vi "front_panel.vi"() -> ()   [LabVIEW 2020]
uses:
  State control.ctl
panel:
  out "Name 2":string
  out "Comments":string
  out "Process":T1
  in  "Status":T2 {"Status - camera" scale=0.0..10.0; "Status - computer" scale=0.0..10.0; "Status - TV" scale=0.0..10.0; "Status - kettle" scale=0.0..10.0; "Status -  microwave" scale=0.0..10.0; "Status - vacuum cleaner" scale=0.0..10.0; "Status - Fridge" scale=0.0..10.0; "Status - washing machine" scale=0.0..10.0}
  in  "Order":T3
  in  "stop":bool
  in  "Adress":string
  in  "Name":string
  in  "OK Button":bool
  # "ORDER"
  # "Warehouse"
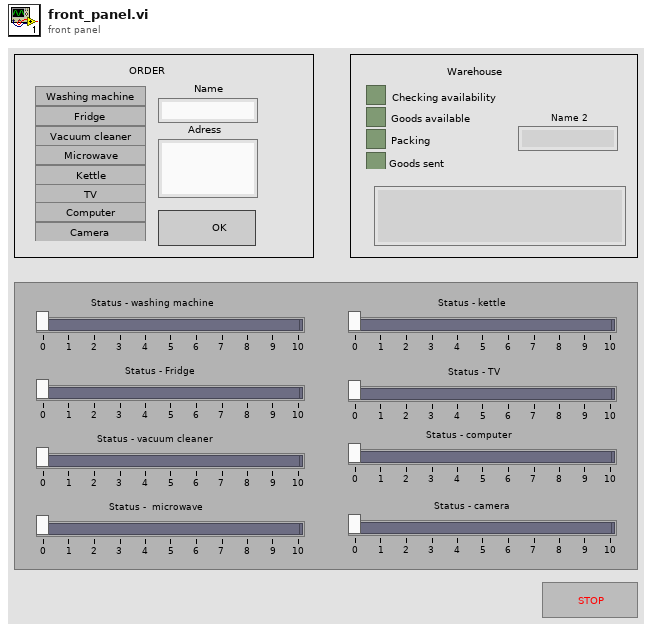
[diagram p1: front panel]
types:
  T1 = cluster{"Checking availability":bool, "Goods available":bool, "Packing":bool, "Goods sent":bool}
  T2 = cluster{"Status - washing machine":u32, "Status - Fridge":u32, "Status - vacuum cleaner":u32, "Status -  microwave":u32, "Status - kettle":u32, "Status - TV":u32, "Status - computer":u32, "Status - camera":u32}
  T3 = cluster{"Washing machine":bool, "Fridge":bool, "Vacuum cleaner":bool, "Microwave":bool, "Kettle":bool, "TV":bool, "Computer":bool, "Camera":bool}
  T4 = typedef "State control.ctl" = enum16{"Init", "avaliability", "goods avaliable", "packing", "sent", "end"}
  T5 = cluster{"Order":cluster{"Washing machine":bool, "Fridge":bool, "Vacuum cleaner":bool, "Microwave":bool, "Kettle":bool, "TV":bool, "Computer":bool, "Camera":bool}, "Adress":string, "Name":string, T4}
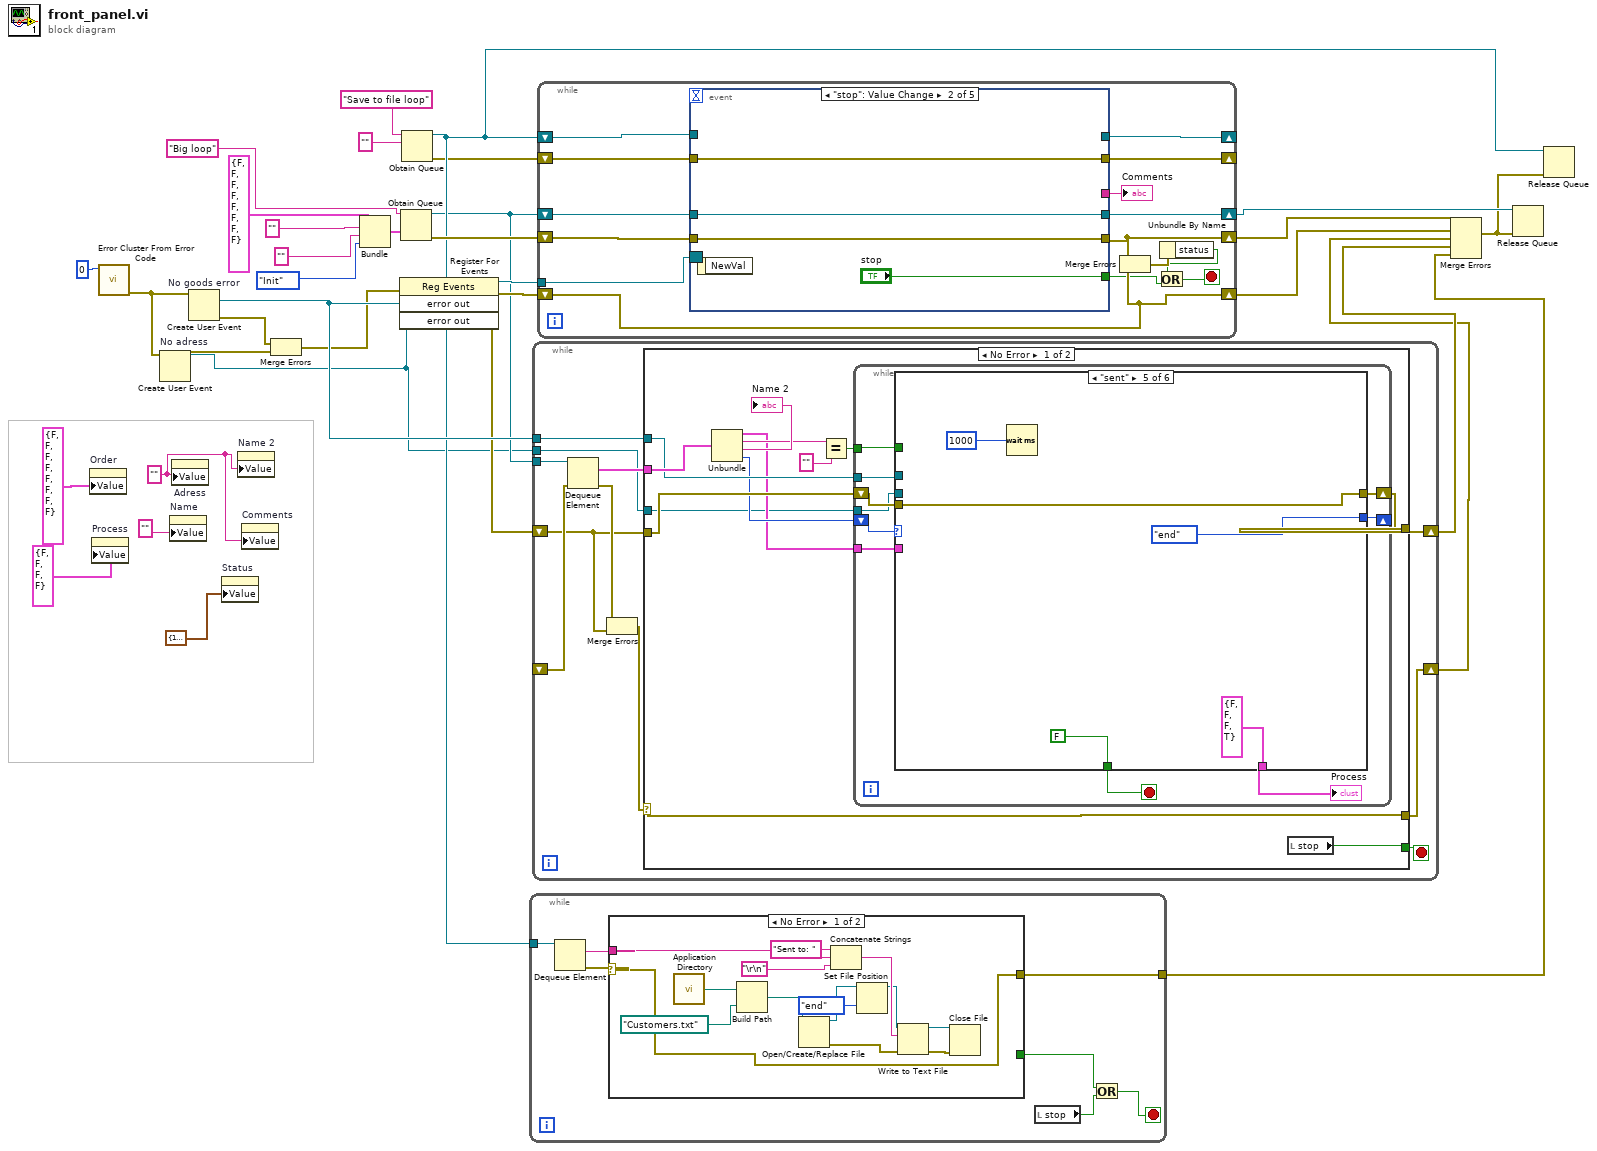
[diagram p0: block diagram]
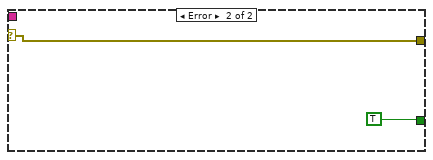
[diagram p2: hidden frame]
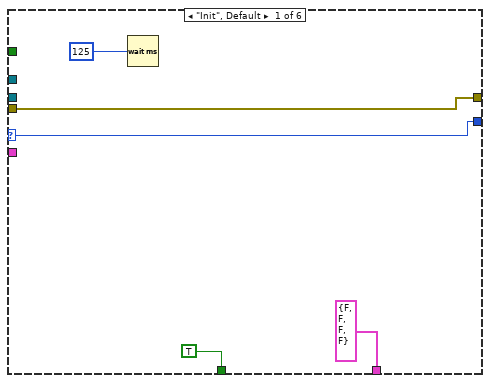
[diagram p3: hidden frame]
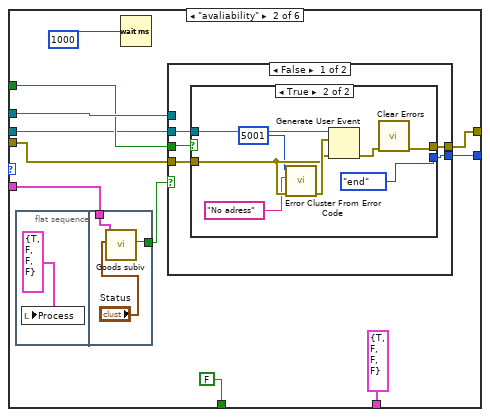
[diagram p4: hidden frame]
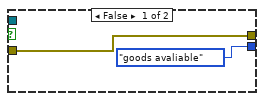
[diagram p5: hidden frame]
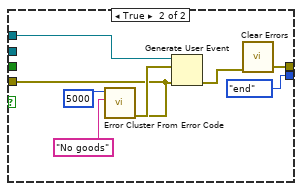
[diagram p6: hidden frame]
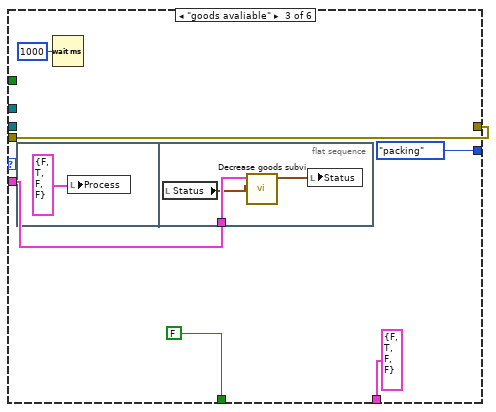
[diagram p7: hidden frame]
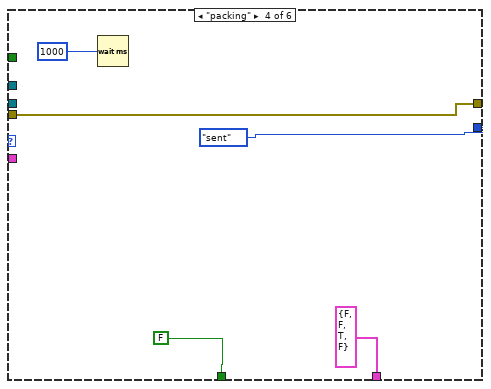
[diagram p8: hidden frame]
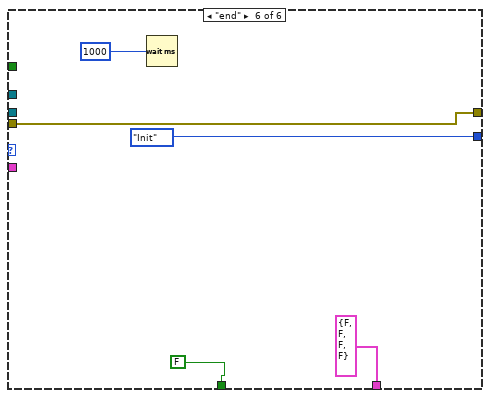
[diagram p9: hidden frame]
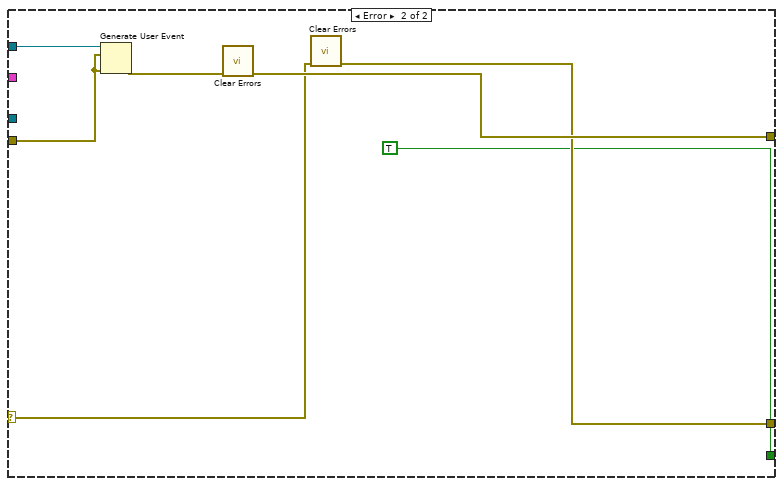
[diagram p10: hidden frame]
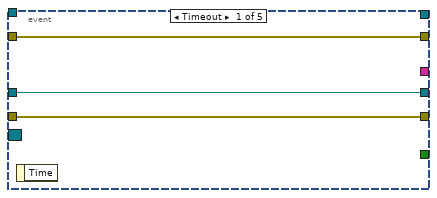
[diagram p11: hidden frame]
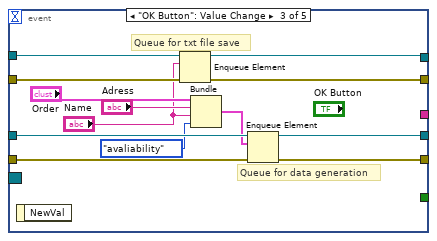
[diagram p12: hidden frame]
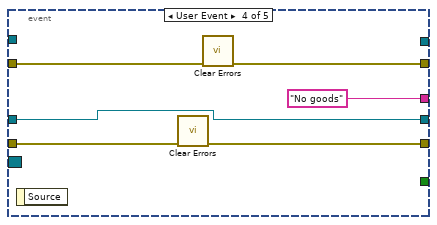
[diagram p13: hidden frame]
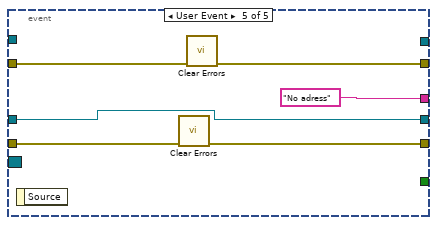
[diagram p14: hidden frame]
diagram:
  w19 = "" ("Adress")
  n1 = property on="Order" class="Clust (strict)"("Value"=T3 {"Washing machine"=FALSE, "Fridge"=FALSE, "Vacuum cleaner"=FALSE, "Microwave"=FALSE, "Kettle"=FALSE, "TV"=FALSE, "Computer"=FALSE, "Camera"=FALSE} ("Order")) -> ()  [unwired: 2 in, 2 out]
  n2 = property on="Process" class="Clust (strict)"("Value"=T1 {"Checking availability"=FALSE, "Goods available"=FALSE, "Packing"=FALSE, "Goods sent"=FALSE} ("Process")) -> ()  [unwired: 2 in, 2 out]
  n3 = call <vilib>:"Error Cluster From Error Code.vi"("error code (0)"=0) -> ("error out"=w9:errorcluster)  [unwired: 8 in]
  n4 = Create User Event "No adress"(user event datatype=w9) -> (user event=w5:refnum<user-event>, error out=w8:errorcluster)  [unwired: 1 in]
  n5 = property on="Name" class="Str"("Value"="" ("Name")) -> ()  [unwired: 2 in, 2 out]
  n6 = property on="Adress" class="Str"("Value"=w19) -> ()  [unwired: 2 in, 2 out]
  n7 = Create User Event "No goods error"(user event datatype=w9) -> (user event=w31:refnum<user-event>, error out=w7:errorcluster)  [unwired: 1 in]
  n8 = property on="Status" class="Clust (strict)"("Value"=T2 {"Status - washing machine"=10, "Status - Fridge"=10, "Status - vacuum cleaner"=10, "Status -  microwave"=10, "Status - kettle"=10, "Status - TV"=10, "Status - computer"=10, "Status - camera"=10} ("Status")) -> ()  [unwired: 2 in, 2 out]
  n9 = property on="Name 2" class="Str"("Value"=w19) -> ()  [unwired: 2 in, 2 out]
  n10 = property on="Comments" class="Str"("Value"=w19) -> ()  [unwired: 2 in, 2 out]
  n11 = Merge Errors(w7, w8) -> (w6:errorcluster)
  n12 = Bundle("Order"=T3 {"Washing machine"=FALSE, "Fridge"=FALSE, "Vacuum cleaner"=FALSE, "Microwave"=FALSE, "Kettle"=FALSE, "TV"=FALSE, "Computer"=FALSE, "Camera"=FALSE}, "Adress"="", "Name"="", State_control."Init") -> (w26:T5)  [unwired: 1 in]
  n13 = register-events(error in=w6, w31, w5) -> (reference out=w32:refnum<event-registration>, error out=w29:errorcluster)  [unwired: 1 in]
  n14 = Obtain Queue(name (unnamed)="Big loop", element data type=w26) -> (queue out=w11:refnum<queue>, error out=w33:errorcluster)  [unwired: 3 in, 1 out]
  n15 = Obtain Queue(name (unnamed)="Save to file loop", element data type="") -> (queue out=w14:refnum<queue>, error out=w13:errorcluster)  [unwired: 3 in, 1 out]
  n16 = while {
    tunnel: w14 -> [w40]
    tunnel: [w34] -> w12
    stop <- w35 stop-if-true
    n17 = Dequeue Element(queue=w40) -> (element=w38:string, error out=w39:errorcluster)  [unwired: 2 in, 2 out]
    n18 = case shown="No Error" w39 {
      selector: w39 -> [w50 w55]
      tunnel: w38 -> [w52 _]
      tunnel: [_ TRUE ("stop")] -> w37
      tunnel: [w50 w55] -> w34
      frame No Error {
        n19 = call <vilib>:"Application Directory.vi"() -> ("Application Directory"=w54:path)
        n20 = Build Path(base path=w54, name or relative path=path "Customers.txt") -> (appended path=w46:path)
        n21 = Open/Create/Replace File(file path (use dialog)=w46) -> (refnum out=w44:refnum<file>, error out=w48:errorcluster)  [unwired: 5 in, 1 out]
        n22 = Concatenate Strings("Sent to: " ("string"), w52, "\r\n") -> (w51:string)
        n23 = Set File Position(refnum=w44, from (0:start)=enum16{"start", "end", "current"}."end") -> (refnum out=w43:refnum<file>)  [unwired: 2 in, 1 out]
        n24 = Write to Text File(file (use dialog)=w43, text=w51, error in=w48) -> (refnum out=w53:refnum<file>, error out=w47:errorcluster)  [unwired: 1 in, 1 out]
        n25 = Close File(refnum=w53, error in=w47) -> ()  [unwired: 2 out]
      }
      frame Error {
      }
    }
    n26 = local read "stop"() -> (w36:bool)
    n27 = Or(x=w37, y=w36) -> (x .or. y?=w35:bool)
  }
  n28 = while {
    tunnel: w11 -> [w67]
    tunnel: w31 -> [w65]
    shift-right: [w59] -> w21
    shift-left: _ -> [w63]
    shift-right: [w62] -> w30
    shift-left: w29 -> [w61]
    tunnel: w5 -> [w57]
    stop <- w58 stop-if-true
    n29 = Dequeue Element(queue=w67, error in (no error)=w63) -> (element=w66:T5, error out=w64:errorcluster)  [unwired: 1 in, 2 out]
    n30 = Merge Errors(w64, w61) -> (w60:errorcluster)
    n31 = case shown="No Error" w60 {
      selector: w60 -> [w80 w161]
      tunnel: w66 -> [w79 _]
      tunnel: w65 -> [w72 w165]
      tunnel: [w73 w162] -> w62
      tunnel: w61 -> [w71 w164]
      tunnel: [w80 w160] -> w59
      tunnel: [w77 TRUE] -> w58
      tunnel: w57 -> [w68 _]
      frame No Error {
        n32 = Unbundle(w79) -> ("Order"=w69:T3, "Adress"=w76:string, "Name"=→"Name 2":string, w70:T4)
        n33 = Equal?(x=w76, y="") -> (x = y?=w74:bool)
        n34 = while {
          tunnel: w74 -> [w89]
          tunnel: w72 -> [w87]
          tunnel: w69 -> [w84]
          shift-right: [w88] -> w73
          shift-left: w71 -> [w86]
          shift-right: [w90] -> _
          shift-left: w70 -> [w85]
          tunnel: w68 -> [w81]
          stop <- w82 stop-if-true
          n35 = case shown="\"sent\"" w85 {
            selector: w85 -> [w91 _ _ _ _ _]
            tunnel: [w91 w104 State_control."packing" State_control."sent" State_control."end" State_control."Init"] -> w90
            tunnel: w89 -> [_ w100 _ _ _ _]
            tunnel: [w95 w101 w138 w148 w153 w158] -> w88
            tunnel: w87 -> [_ w103 _ _ _ _]
            tunnel: w86 -> [w95 w102 w138 w148 w153 w158]
            tunnel: w84 -> [_ w99 w134 _ _ _]
            tunnel: [T1 {"Checking availability"=FALSE, "Goods available"=FALSE, "Packing"=FALSE, "Goods sent"=FALSE} ("Process") T1 {"Checking availability"=TRUE, "Goods available"=FALSE, "Packing"=FALSE, "Goods sent"=FALSE} ("Process") T1 {"Checking availability"=FALSE, "Goods available"=TRUE, "Packing"=FALSE, "Goods sent"=FALSE} ("Process") T1 {"Checking availability"=FALSE, "Goods available"=FALSE, "Packing"=TRUE, "Goods sent"=FALSE} ("Process") T1 {"Checking availability"=FALSE, "Goods available"=FALSE, "Packing"=FALSE, "Goods sent"=TRUE} ("Process") T1 {"Checking availability"=FALSE, "Goods available"=FALSE, "Packing"=FALSE, "Goods sent"=FALSE} ("Process")] -> w83
            tunnel: [TRUE FALSE FALSE FALSE FALSE FALSE] -> w82
            tunnel: w81 -> [_ w96 _ _ _ _]
            frame "Init", Default {
              n36 = Wait (ms)(milliseconds to wait=u32 125) -> ()  [unwired: 1 out]
            }
            frame "avaliability" {
              n37 = flat-sequence {
                tunnel: w99 -> [w110]
                tunnel: [w109] -> w98
                frame #0 {
                  n38 = local write "Process"(T1 {"Checking availability"=TRUE, "Goods available"=FALSE, "Packing"=FALSE, "Goods sent"=FALSE} ("Process")) -> ()
                }
                frame #1 {
                  n39 = call "Goods subiv.vi"("Status"="Status", "Order"=w110) -> ("avalibity"=w109:bool)  [unwired: 7 in]
                }
              }
              n40 = Wait (ms)(milliseconds to wait=u32 1000) -> ()  [unwired: 1 out]
              n41 = case shown="False" w98 {
                tunnel: [w114 State_control."end"] -> w104
                tunnel: w103 -> [_ w132]
                tunnel: w102 -> [w113 w129]
                tunnel: [w112 w126] -> w101
                tunnel: w100 -> [w115 _]
                tunnel: w96 -> [w111 _]
                frame False {
                  n42 = case shown="True" w115 {
                    tunnel: [State_control."goods avaliable" State_control."end"] -> w114
                    tunnel: w113 -> [w116 w123]
                    tunnel: [w116 w118] -> w112
                    tunnel: w111 -> [_ w120]
                    frame False {
                    }
                    frame True {
                      n43 = call <vilib>:"Error Cluster From Error Code.vi"("error in (no error)"=w123, "error message (\"\")"="No adress", "error code (0)"=5001) -> ("error out"=w124:errorcluster)  [unwired: 6 in]
                      n44 = Generate User Event(user event=w120, event data cluster=w124, error in=w123) -> (error out=w119:errorcluster)  [unwired: 1 in, 1 out]
                      n45 = call <vilib>:"Clear Errors.vi"("error in (no error)"=w119) -> ("error out"=w118:errorcluster)  [unwired: 5 in, 1 out]
                    }
                  }
                }
                frame True {
                  n46 = call <vilib>:"Error Cluster From Error Code.vi"("error in (no error)"=w129, "error message (\"\")"="No goods", "error code (0)"=5000) -> ("error out"=w131:errorcluster)  [unwired: 6 in]
                  n47 = Generate User Event(user event=w132, event data cluster=w131, error in=w129) -> (error out=w127:errorcluster)  [unwired: 1 in, 1 out]
                  n48 = call <vilib>:"Clear Errors.vi"("error in (no error)"=w127) -> ("error out"=w126:errorcluster)  [unwired: 5 in, 1 out]
                }
              }
            }
            frame "goods avaliable" {
              n49 = flat-sequence {
                tunnel: w134 -> [w143]
                frame #0 {
                  n50 = local write "Process"(T1 {"Checking availability"=FALSE, "Goods available"=TRUE, "Packing"=FALSE, "Goods sent"=FALSE} ("Process")) -> ()
                }
                frame #1 {
                  n51 = local read "Status"() -> (w142:T2)
                  n52 = call "Decrease goods subvi.vi"("Status"=w142, "Order"=w143) -> ("Cluster"=w141:T2)  [unwired: 9 in]
                  n53 = local write "Status"(w141) -> ()
                }
              }
              n54 = Wait (ms)(milliseconds to wait=u32 1000) -> ()  [unwired: 1 out]
            }
            frame "packing" {
              n55 = Wait (ms)(milliseconds to wait=u32 1000) -> ()  [unwired: 1 out]
            }
            frame "sent" {
              n56 = Wait (ms)(milliseconds to wait=u32 1000) -> ()  [unwired: 1 out]
            }
            frame "end" {
              n57 = Wait (ms)(milliseconds to wait=u32 1000) -> ()  [unwired: 1 out]
            }
          }
          "Process" <- w83
        }
        n58 = local read "stop"() -> (w77:bool)
      }
      frame Error {
        n59 = Generate User Event(user event=w165, event data cluster=w164, error in=w164) -> (error out=w163:errorcluster)  [unwired: 1 in, 1 out]
        n60 = call <vilib>:"Clear Errors.vi"("error in (no error)"=w163) -> ("error out"=w162:errorcluster)  [unwired: 5 in, 1 out]
        n61 = call <vilib>:"Clear Errors.vi"("error in (no error)"=w161) -> ("error out"=w160:errorcluster)  [unwired: 5 in, 1 out]
      }
    }
  }
  n62 = while {
    shift-right: [w171] -> w27
    shift-left: w33 -> [w166]
    tunnel: w32 -> [w174]
    shift-right: [w172] -> w28
    shift-left: w29 -> [w172]
    shift-right: [w179] -> w2
    shift-left: w11 -> [w180]
    shift-right: [w177] -> _
    shift-left: w14 -> [w178]
    shift-right: [w175] -> _
    shift-left: w13 -> [w176]
    stop <- w168 stop-if-true
    n63 = event shown="[1] \"stop\": Value Change" {
      selector: w174 -> [_ _ _ _ _]
      dyn-events: _ -> [_ _ _ _ _]
      timeout: _ -> [_ _ _ _ _]
      tunnel: [_ "stop" _ _ _] -> w167
      tunnel: w180 -> [w181 w184 w200 w201 w207]
      tunnel: w166 -> [w182 w186 w199 w205 w211]
      tunnel: [w182 w186 w188 w202 w210] -> w171
      tunnel: [w181 w184 w194 w201 w207] -> w179
      tunnel: w178 -> [_ _ w193 _ _]
      tunnel: [_ _ w192 _ _] -> w177
      tunnel: w176 -> [w183 w185 w191 w204 w209]
      tunnel: [w183 w185 w190 w203 w208] -> w175
      tunnel: [_ _ _ "No goods" ("Comments") "No adress" ("Comments")] -> w173
      event Timeout {
        n64 = event-data() -> ()  [unwired: 1 in, 1 out]
      }
      event "stop": Value Change {
        n65 = event-data() -> ()  [unwired: 1 in, 1 out]
      }
      event "OK Button": Value Change {
        # "Queue for data generation"
        # "Queue for txt file save"
        n66 = event-data() -> ()  [unwired: 1 in, 1 out]
        n67 = Enqueue Element(queue=w193, element="Name", error in (no error)=w191) -> (queue out=w192:refnum<queue>, error out=w190:errorcluster)  [unwired: 1 in, 1 out]
        n68 = Bundle("Order"="Order", "Adress"="Adress", "Name"="Name", State_control."avaliability") -> (w195:T5)  [unwired: 1 in]
        n69 = Enqueue Element(queue=w200, element=w195, error in (no error)=w199) -> (queue out=w194:refnum<queue>, error out=w188:errorcluster)  [unwired: 1 in, 1 out]
      }
      event User Event {
        n70 = event-data() -> ()  [unwired: 1 in, 1 out]
        n71 = call <vilib>:"Clear Errors.vi"("error in (no error)"=w205) -> ("error out"=w202:errorcluster)  [unwired: 5 in, 1 out]
        n72 = call <vilib>:"Clear Errors.vi"("error in (no error)"=w204) -> ("error out"=w203:errorcluster)  [unwired: 5 in, 1 out]
      }
      event User Event {
        n73 = event-data() -> ()  [unwired: 1 in, 1 out]
        n74 = call <vilib>:"Clear Errors.vi"("error in (no error)"=w211) -> ("error out"=w210:errorcluster)  [unwired: 5 in, 1 out]
        n75 = call <vilib>:"Clear Errors.vi"("error in (no error)"=w209) -> ("error out"=w208:errorcluster)  [unwired: 5 in, 1 out]
      }
    }
    "Comments" <- w173
    n76 = Merge Errors(w171, w172) -> (w170:errorcluster)
    n77 = Unbundle By Name(w170) -> ("status"=w169:bool)
    n78 = Or(x=w169, y=w167) -> (x .or. y?=w168:bool)
  }
  n79 = Merge Errors(w27, w28, w21, w30, w12) -> (w1:errorcluster)
  n80 = Release Queue(queue=w2, error in (no error)=w1) -> ()  [unwired: 1 in, 3 out]
  n81 = Release Queue(queue=w14, error in (no error)=w1) -> ()  [unwired: 1 in, 3 out]
